vi "compatFileDialog.vi"(4 "pattern label":string, 5 "button label":string, 7 "prompt":string, 8 "pattern":string, 9 "default name":string, 10 "select mode (2)":T1(ring)=enum."new or existing file", 11 "start path":path=path "") -> (0 "cancelled":bool, 1 "exists":bool, 2 "path":path)   [LabVIEW 2020]
doc: "Compatibility VI for the LabVIEW 7.1 File Dialog to keep functionality when a non-constant is wired into the select mode input."
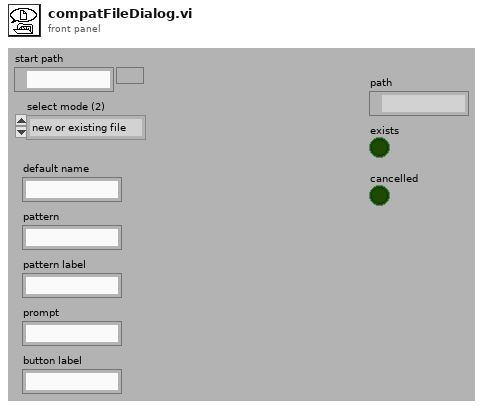
[diagram p1: front panel]
types:
  T1 = enum32{"existing file", "new file", "new or existing file", "existing dir", "new dir", "new or existing dir", "existing file (use LLBs)", "new file (use LLBs)", "new or existing file (use LLBs)", "new or existing file or directory (use LLBs)"}
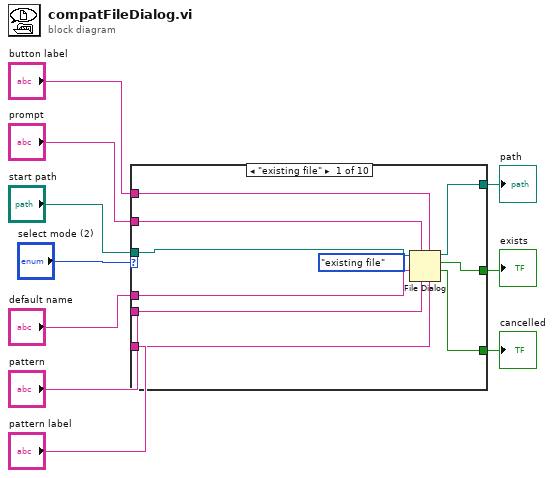
[diagram p0: block diagram]
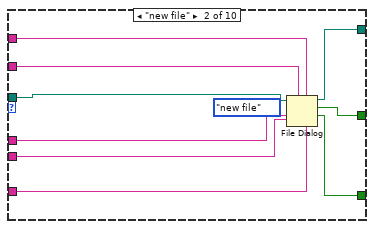
[diagram p2: hidden frame]
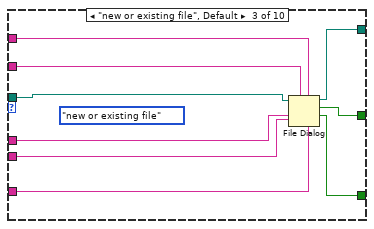
[diagram p3: hidden frame]
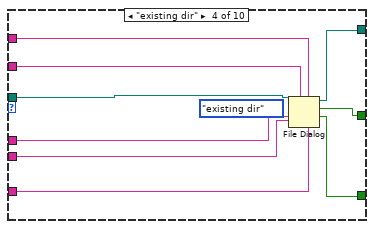
[diagram p4: hidden frame]
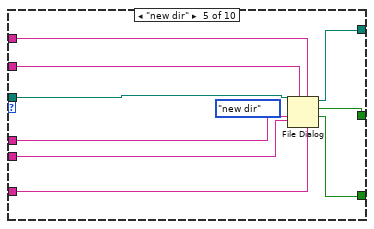
[diagram p5: hidden frame]
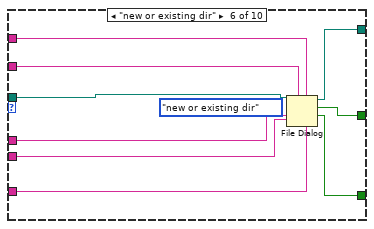
[diagram p6: hidden frame]
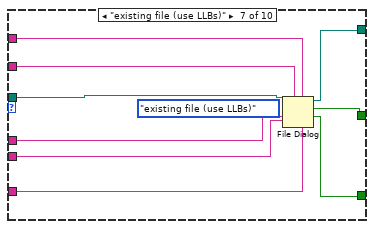
[diagram p7: hidden frame]
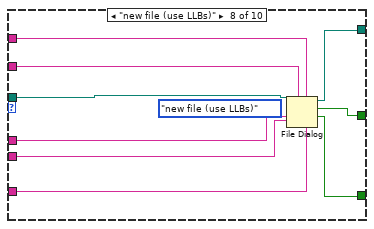
[diagram p8: hidden frame]
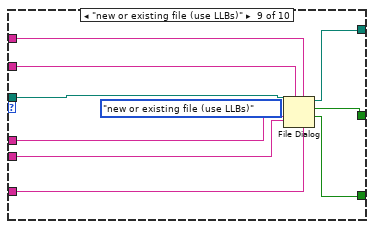
[diagram p9: hidden frame]
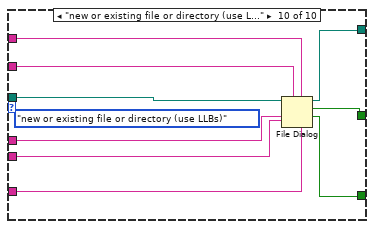
[diagram p10: hidden frame]
diagram:
  n1 = case shown="\"existing file\"" "select mode (2)" {
    tunnel: "start path" -> [w11 w20 w29 w38 w47 w56 w65 w74 w83 w92]
    tunnel: "default name" -> [w14 w23 w30 w41 w50 w59 w68 w77 w86 w95]
    tunnel: "pattern" -> [w13 w24 w31 w40 w51 w60 w69 w76 w85 w94]
    tunnel: "pattern label" -> [w12 w25 w32 w39 w52 w61 w70 w75 w84 w93]
    tunnel: "prompt" -> [w15 w22 w34 w42 w49 w58 w67 w78 w87 w96]
    tunnel: "button label" -> [w16 w21 w33 w43 w48 w57 w66 w79 w88 w97]
    tunnel: [w17 w27 w37 w44 w55 w64 w73 w80 w89 w98] -> w3
    tunnel: [w18 w28 w36 w45 w54 w63 w72 w81 w90 w99] -> w2
    tunnel: [w19 w26 w35 w46 w53 w62 w71 w82 w91 w100] -> w1
    frame "existing file" {
      (unwired) T1."existing file" ("select mode (2)")
      n2 = File Dialog(4:w12, 5:w16, 6:w13, 7:w15, 9:w14, 11:w11) -> (1:w19:bool, 2:w18:bool, 3:w17:path)  [unwired: 1 in, 1 out]
    }
    frame "new file" {
      (unwired) T1."new file" ("select mode (2)")
      n3 = File Dialog(4:w25, 5:w21, 6:w24, 7:w22, 9:w23, 11:w20) -> (1:w26:bool, 2:w28:bool, 3:w27:path)  [unwired: 1 in, 1 out]
    }
    frame "new or existing file", Default {
      (unwired) T1."new or existing file" ("select mode (2)")
      n4 = File Dialog(4:w32, 5:w33, 6:w31, 7:w34, 9:w30, 11:w29) -> (1:w35:bool, 2:w36:bool, 3:w37:path)  [unwired: 1 in, 1 out]
    }
    frame "existing dir" {
      (unwired) T1."existing dir" ("select mode (2)")
      n5 = File Dialog(4:w39, 5:w43, 6:w40, 7:w42, 9:w41, 11:w38) -> (1:w46:bool, 2:w45:bool, 3:w44:path)  [unwired: 1 in, 1 out]
    }
    frame "new dir" {
      (unwired) T1."new dir" ("select mode (2)")
      n6 = File Dialog(4:w52, 5:w48, 6:w51, 7:w49, 9:w50, 11:w47) -> (1:w53:bool, 2:w54:bool, 3:w55:path)  [unwired: 1 in, 1 out]
    }
    frame "new or existing dir" {
      (unwired) T1."new or existing dir" ("select mode (2)")
      n7 = File Dialog(4:w61, 5:w57, 6:w60, 7:w58, 9:w59, 11:w56) -> (1:w62:bool, 2:w63:bool, 3:w64:path)  [unwired: 1 in, 1 out]
    }
    frame "existing file (use LLBs)" {
      (unwired) T1."existing file (use LLBs)" ("select mode (2)")
      n8 = File Dialog(4:w70, 5:w66, 6:w69, 7:w67, 9:w68, 11:w65) -> (1:w71:bool, 2:w72:bool, 3:w73:path)  [unwired: 1 in, 1 out]
    }
    frame "new file (use LLBs)" {
      (unwired) T1."new file (use LLBs)" ("select mode (2)")
      n9 = File Dialog(4:w75, 5:w79, 6:w76, 7:w78, 9:w77, 11:w74) -> (1:w82:bool, 2:w81:bool, 3:w80:path)  [unwired: 1 in, 1 out]
    }
    frame "new or existing file (use LLBs)" {
      (unwired) T1."new or existing file (use LLBs)" ("select mode (2)")
      n10 = File Dialog(4:w84, 5:w88, 6:w85, 7:w87, 9:w86, 11:w83) -> (1:w91:bool, 2:w90:bool, 3:w89:path)  [unwired: 1 in, 1 out]
    }
    frame "new or existing file or directory (use LLBs)" {
      (unwired) T1."new or existing file or directory (use LLBs)" ("select mode (2)")
      n11 = File Dialog(4:w93, 5:w97, 6:w94, 7:w96, 9:w95, 11:w92) -> (1:w100:bool, 2:w99:bool, 3:w98:path)  [unwired: 1 in, 1 out]
    }
  }
  "path" <- w3
  "exists" <- w2
  "cancelled" <- w1
